vi "Raycaster_FizzleFade.vi"(11 "Frame Buffers In":T1) -> (3 "Frame Buffers Out":T1)   [LabVIEW 2020]
uses:
  Controls/Raycaster_DrawState.ctl
  <vilib>/rvi/DataTransferAndStorage/Container/XNode/niFpgaContainer.xnode
  <vilib>/rvi/DataTransferAndStorage/Register/Emulation/niFpgaRegisterEmulation.vi
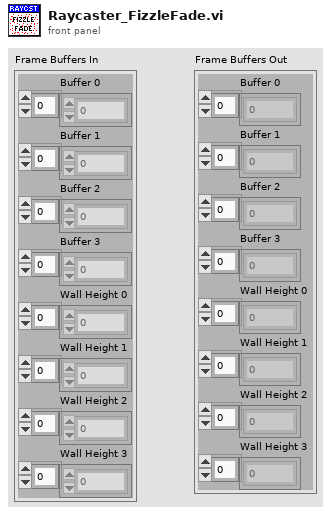
[diagram p1: front panel]
types:
  T1 = typedef "Raycaster_DrawState.ctl" = cluster{"Buffer 0":u8[], "Buffer 1":u8[], "Buffer 2":u8[], "Buffer 3":u8[], "Wall Height 0":i16[], "Wall Height 1":i16[], "Wall Height 2":i16[], "Wall Height 3":i16[]}
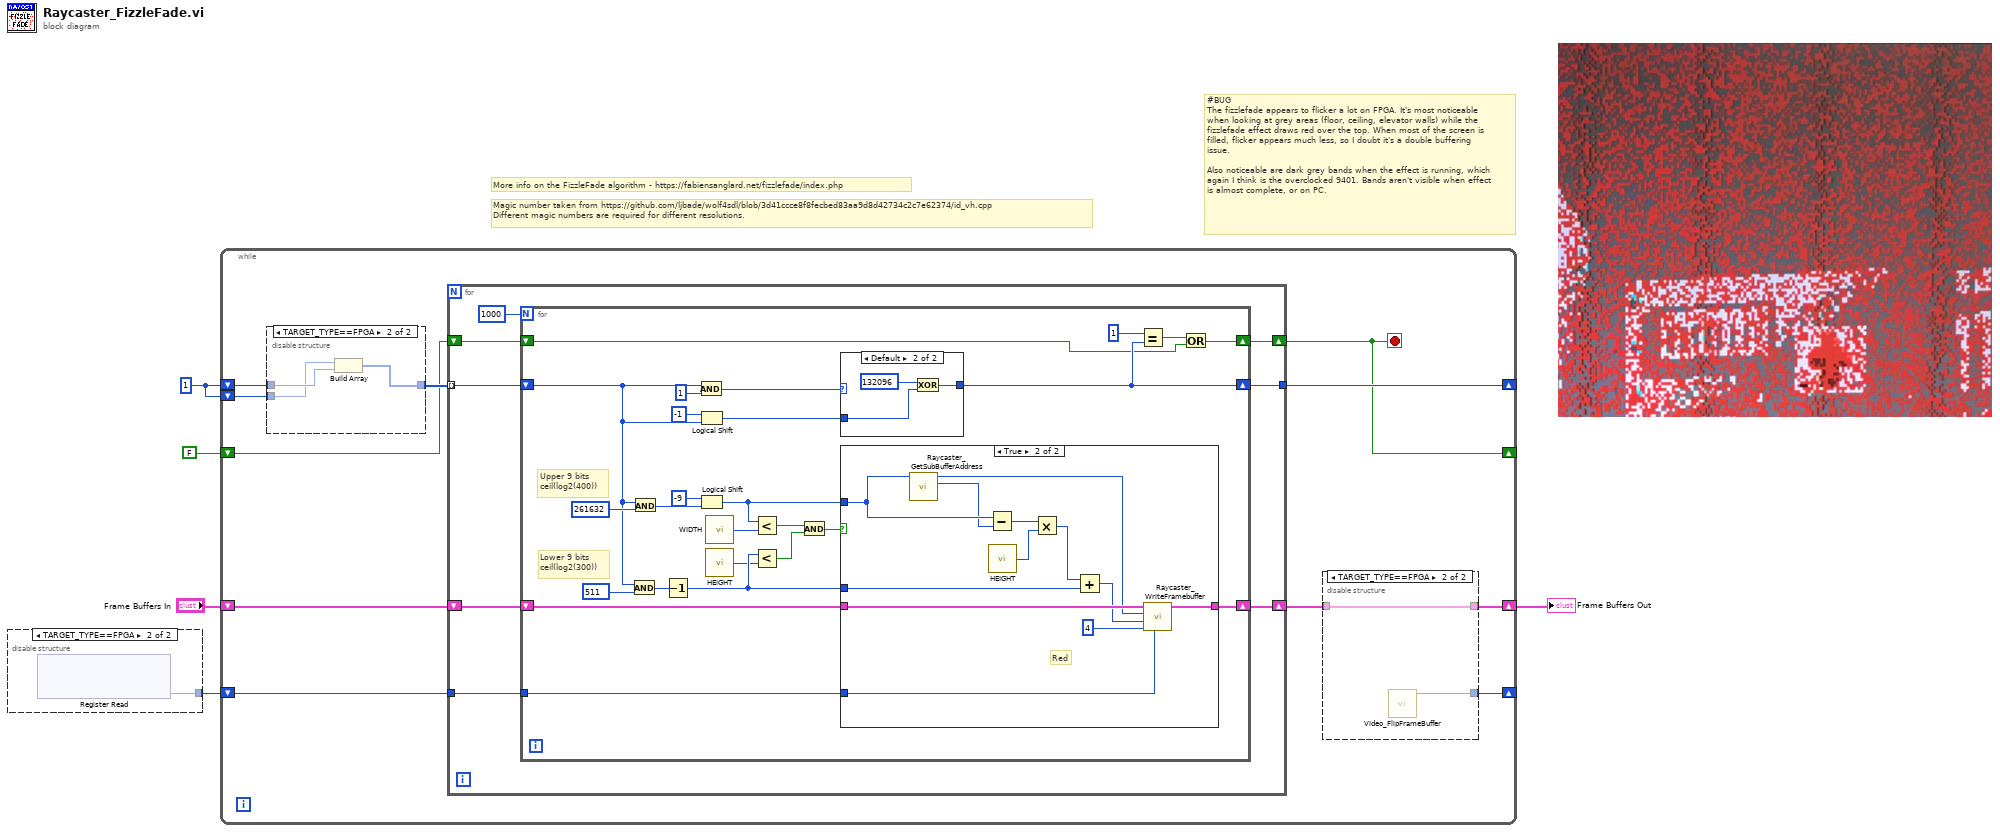
[diagram p0: block diagram]
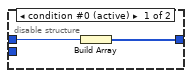
[diagram p2: hidden frame]
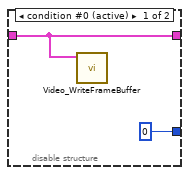
[diagram p5: hidden frame]
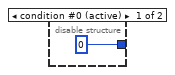
[diagram p6: hidden frame]
diagram:
  w5 = u32 1
  # "#BUG\nThe fizzlefade appears to flicker a lot on FPGA. It's most noticeable when looking at grey areas (floor, ceiling, elevator walls) while the fizzlefade effect draws red over the top. When most of the screen is filled, flicker appears much less, so I doubt it's a double buffering issue.\n\nAlso noticeable are dark grey bands when the effect is running, which again I think is the overclocked 9401. Bands aren't visible when effect is almost complete, or on PC."
  # "More info on the FizzleFade algorithm - https://fabiensanglard.net/fizzlefade/index.php"
  # "Magic number taken from https://github.com/ljbade/wolf4sdl/blob/3d41ccce8f8fecbed83aa9d8d42734c2c7e62374/id_vh.cpp\nDifferent magic numbers are required for different resolutions."
  n1 = disable-structure "Conditional Disable Structure" shown="TARGET_TYPE==FPGA" {
    disable-tunnel: [u8 0 ("Data") w7] -> w3
    frame condition #0 (active) {
    }
    frame condition #1 {
      n2 = xnode ("Register Read")() -> ("Data"=w7:u8)  [unwired: 1 in, 1 out]
    }
  }
  n3 = while {
    shift-right: [w18] -> _
    shift-left: w5 -> [w14]
    shift-right: [w15] -> w1
    shift-left: "Frame Buffers In" -> [w17]
    shift-left: w5 -> [w13]
    shift-right: [w10] -> _
    shift-left: FALSE -> [w11]
    shift-right: [w8] -> _
    shift-left: w3 -> [w9]
    stop <- w10 stop-if-true
    n4 = disable-structure "Conditional Disable Structure" shown="TARGET_TYPE==FPGA" {
      disable-tunnel: w14 -> [w20 w23]
      disable-tunnel: w13 -> [_ w22]
      disable-tunnel: [w19 w21] -> w12
      frame condition #0 (active) {
        n5 = Build Array(w20) -> (w19:u32[])
      }
      frame condition #1 {
        n6 = Build Array(w22, w23) -> (w21:u32[])
      }
    }
    n7 = for {
      tunnel: w12 -> [w31] mode=indexing
      tunnel: [w30] -> w18
      tunnel: w9 -> [w26]
      shift-right: [w28] -> w16
      shift-left: w17 -> [w29]
      shift-right: [w25] -> w10
      shift-left: w11 -> [w24]
      n8 = for {
        N: 1000 -> [_]
        shift-right: [w38] -> w28
        shift-left: w29 -> [w39]
        shift-right: [w36] -> w30
        shift-left: w31 -> [w50]
        tunnel: w26 -> [w37]
        shift-right: [w33] -> w25
        shift-left: w24 -> [w32]
        # "Upper 9 bits\nceil(log2(400))"
        # "Lower 9 bits\nceil(log2(300))"
        n9 = And(x=w50, y=u32 511) -> (x .and. y?=w44:u32)
        n10 = And(x=w50, y=u32 261632) -> (x .and. y?=w54:u32)
        n11 = Decrement(x=w44) -> (x-1=w42:u32)
        n12 = And(x=w50, y=u32 1) -> (x .and. y?=w49:u32)
        n13 = Logical Shift(y=i16 -1, x=w50) -> (x << y=w48:u32)
        n14 = Logical Shift(y=i16 -9, x=w54) -> (x << y=w43:u32)
        n15 = call "WIDTH.vi"() -> ("WIDTH"=w40:i16)
        n16 = call "HEIGHT.vi"() -> ("HEIGHT"=w41:i16)
        n17 = Less?(x=w43, y=w40) -> (x < y?=w46:bool)
        n18 = Less?(x=w42, y=w41) -> (x < y?=w47:bool)
        n19 = And(x=w46, y=w47) -> (x .and. y?=w45:bool)
        n20 = case shown="Default" w49 {
          tunnel: w48 -> [w57 w60]
          tunnel: [w57 w58] -> w36
          frame 0 {
          }
          frame Default {
            n21 = Exclusive Or(1:w60, 2:u32 132096 ("y")) -> (0:w58:u32)
          }
        }
        n22 = case shown="True" w45 {
          tunnel: w42 -> [_ w70]
          tunnel: w43 -> [_ w69]
          tunnel: w39 -> [w61 w67]
          tunnel: [w61 w62] -> w38
          tunnel: w37 -> [_ w63]
          frame False {
          }
          frame True {
            # "Red"
            n23 = call "Raycaster_GetSubBufferAddress.vi"("Column"=w69) -> ("Start Address"=w68:i16, "Sub Buffer"=w66:u8)  [unwired: 9 in]
            n24 = Subtract(x=w69, y=w68) -> (x-y=w73:u32)
            n25 = call "HEIGHT.vi"() -> ("HEIGHT"=w72:i16)
            n26 = Multiply(x=w73, y=w72) -> (x*y=w71:u32)
            n27 = Add(x=w71, y=w70) -> (x+y=w64:u32)
            n28 = call "Raycaster_WriteFramebuffer.vi"("Offscreen Buffer"=w63, "Value"=u8 4 ("new element/subarray"), "Sub Buffer Address"=w64, "Sub Buffer"=w66, "Frame Buffers In"=w67) -> ("Frame Buffers Out"=w62:T1)  [unwired: 6 in]
          }
        }
        n29 = Equal?(x=u32 1 ("y"), y=w36) -> (x = y?=w34:bool)
        n30 = Or(x=w34, y=w32) -> (x .or. y?=w33:bool)
      }
    }
    n31 = disable-structure "Conditional Disable Structure" shown="TARGET_TYPE==FPGA" {
      disable-tunnel: w16 -> [w74 w77]
      disable-tunnel: [w74 w77] -> w15
      disable-tunnel: [u8 0 ("Data") w76] -> w8
      frame condition #0 (active) {
        n32 = call "Video_WriteFrameBuffer.vi"("Frame Buffers"=w74) -> ()  [unwired: 10 in, 1 out]
      }
      frame condition #1 {
        n33 = call "Video_FlipFrameBuffer.vi"() -> ("New Offscreen Buffer"=w76:u8)  [unwired: 11 in]
      }
    }
  }
  "Frame Buffers Out" <- w1
